vi "Set GUI Control.vi"(8 "error in (no error)":errorcluster, 10 "GUI Control":refnum<class "GUI Control.lvclass">, 11 "Add Control_Behavior in":refnum<class "Add Control_Behavior.lvclass">) -> (0 "error out":errorcluster, 3 "Add Control_Behavior out":refnum<class "Add Control_Behavior.lvclass">)   [LabVIEW 2015, in "Add Control_Behavior.lvclass"]
uses:
  Add Control_Behavior.lvclass
  GUI/GUI Controls/GUI Control/GUI Control.lvclass
  Add Control_Behavior.lvclass/Add Control_Behavior.ctl
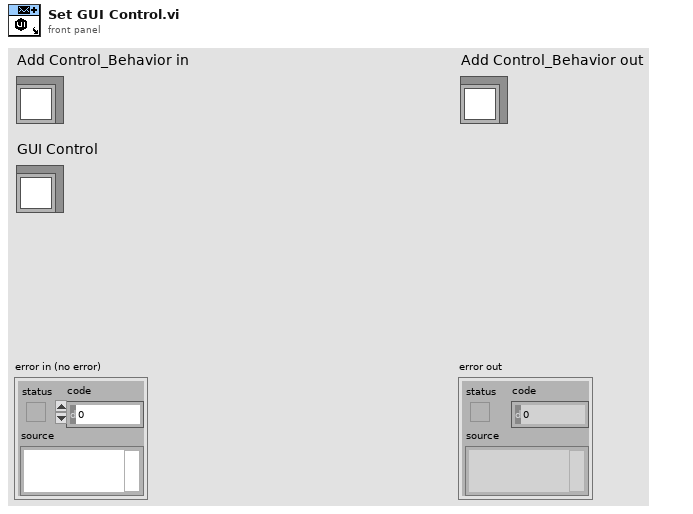
[diagram p1: front panel]
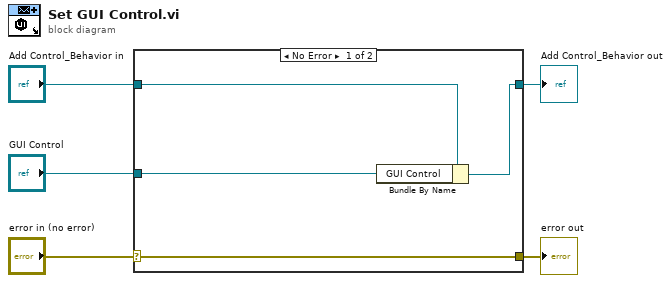
[diagram p0: block diagram]
diagram:
  n1 = case shown="No Error" "error in (no error)" {
    selector: "error in (no error)" -> [w9 w10]
    tunnel: [w9 w10] -> w4
    tunnel: [w7 w11] -> w2
    tunnel: "Add Control_Behavior in" -> [w8 w11]
    tunnel: "GUI Control" -> [w6 _]
    frame No Error {
      n2 = Bundle By Name(cluster=w8, "GUI Control"=w6) -> (w7:refnum<class "Add Control_Behavior.lvclass">)
    }
    frame Error {
    }
  }
  "error out" <- w4
  "Add Control_Behavior out" <- w2
